vi "dfd_Convert DataType to Representation.vi"(4 "data type":T1 items=["I16", "I32"]) -> (1 "representation":T2(ring))   [LabVIEW 2017, in "NI_DigFilterLicensed.lvlib"]
uses:
  <vilib>/addons/Digital Filter Design/NI_DigFilterLicensed.lvlib
  <vilib>/addons/Digital Filter Design/_Objects.llb/DFD Multirate Coef Type.ctl
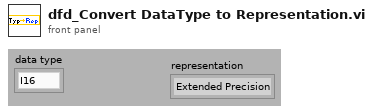
[diagram p1: front panel]
types:
  T1 = typedef "NI_DigFilterLicensed.lvlib/DFD Multirate Coef Type.ctl" = u16
  T2 = enum32{"Extended Precision", "Double Precision", "Single Precision", "Long", "Word", "Byte", "Unsigned Long", "Unsigned Word", "Unsigned Byte", "Complex Extended", "Complex Double", "Complex Single", "Quad", "Unsigned Quad"}
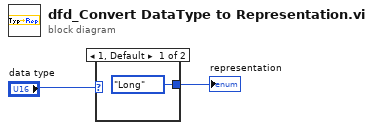
[diagram p0: block diagram]
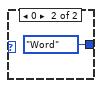
[diagram p2: hidden frame]
diagram:
  n1 = case shown="1, Default" "data type" {
    tunnel: [T2."Long" ("new representation") T2."Word" ("new representation")] -> w2
    frame 1, Default {
    }
    frame 0 {
    }
  }
  "representation" <- w2
